vi "S7_ReadBool.vi"(7 "address":string, 8 "错误输入":errorcluster caption="错误输入（无错误）", 11 "connect id":refnum<k24>) -> (0 "错误输出":errorcluster, 1 "value":bool, 2 "IsSuccess":bool, 3 "connect id":refnum<k24>)   [LabVIEW 2018]
uses:
  E:/Fergus/S7/S7_code/Lib/HslCommunication.dll
  Lib/HslCommunication.dll
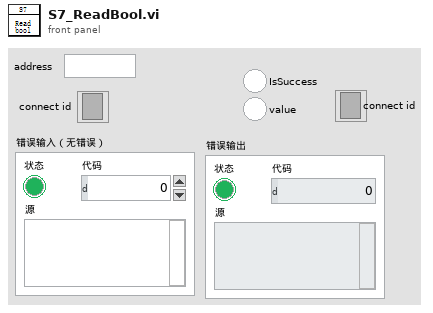
[diagram p1: front panel]
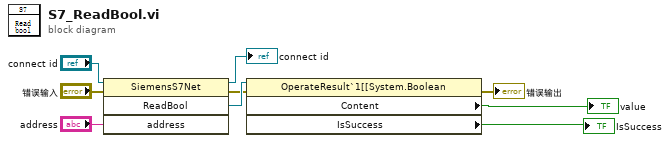
[diagram p0: block diagram]
diagram:
  n1 = invoke on="调用节点" class="SiemensS7Net" method="ReadBool"(reference="connect id", error in="错误输入", "address"="address") -> (reference out=→"connect id":refnum<k24>, error out=w5:errorcluster, "ReadBool"=w6:refnum<k24>)  [unwired: 1 in, 1 out]
  n2 = property class="OperateResult`1[[System.Boolean"(reference=w6, error in=w5) -> (error out=→"错误输出":errorcluster, "Content"=→"value":bool, "IsSuccess"=→"IsSuccess":bool)  [unwired: 1 out]
